vi "Mix Secret Number.vi"(10 "Value":u64, 11 "Current Secret Number":u64) -> (3 "New Secret Number":u64)   [LabVIEW 2024]
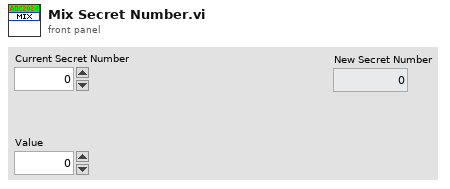
[diagram p1: front panel]
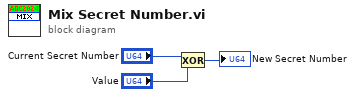
[diagram p0: block diagram]
diagram:
  n1 = Exclusive Or(1:"Value", 2:"Current Secret Number") -> (0:→"New Secret Number":u64)
